vi "WPI_CameraSetScaledAttr_EDIT.vi"(7 "Attr Format":string="CameraAttributes::%s::Value", 8 "error in (no error)":errorcluster, 9 "Scaled":dbl, 10 "Attr String":string, 11 "Camera Address In":string) -> (0 "error out":errorcluster, 3 "Camera Address Out":string)   [LabVIEW 2015]
doc: "This VI updates an attribute where input unit is percentage and camera parameter may be in another unit.\n\nThis software is licensed. Open the labview\\readme\\WPI Robotics Library Open Source License.txt file for more information."
uses:
  <vilib>/userdefined/High Color/IMAQdx.ctl
  <resource>/objmgr/imaqdx.rc
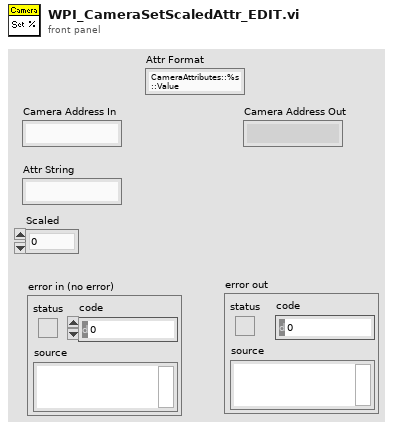
[diagram p1: front panel]
types:
  T1 = typedef "IMAQdx.ctl" = refnum<k21>
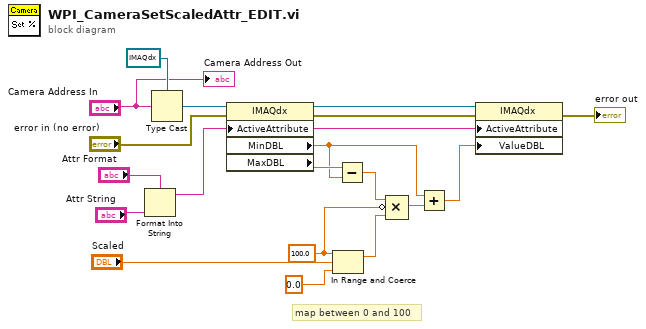
[diagram p0: block diagram]
diagram:
  w10 = 100.0
  # "map between 0 and 100"
  n1 = Format Into String(format string="Attr Format", "Attr String") -> (resulting string=w5:string)  [unwired: 2 in, 1 out]
  n2 = Type Cast(type=T1 refnum ("Session In"), x="Camera Address In") -> (*(type *) &x=w18:T1)
  n3 = property class="IMAQdx"(reference=w18, error in="error in (no error)", "ActiveAttribute"=w5) -> (reference out=w6:T1, error out=w2:errorcluster, "MinDBL"=w7:dbl, "MaxDBL"=w14:dbl)
  n4 = In Range and Coerce(upper limit=w10, x="Scaled", lower limit=0.0) -> (coerced(x)=w9:dbl)  [unwired: 1 out]
  n5 = Subtract(x=w14, y=w7) -> (x-y=w13:dbl)
  n6 = Compound Arithmetic op=MULTIPLY(w13, invert w10, w9) -> (w8:dbl)
  n7 = Add(x=w7, y=w8) -> (x+y=w4:dbl)
  n8 = property class="IMAQdx"(reference=w6, error in=w2, "ActiveAttribute"=w5, "ValueDBL"=w4) -> (error out=→"error out":errorcluster)  [unwired: 1 out]
  "Camera Address Out" <- "Camera Address In"
